vi "ge_PopGlobals.vi"(8 "error in":errorcluster, 9 "Selected Rows":i32[](array[numeric]), 10 "ChanGrp.lvclass":refnum<class "ChanGrp.lvclass">, 11 "ge_DAQManDefinitions":T1) -> (0 "error out":errorcluster, 1 "DefVal":u16=65535, 3 "Ring Support For Group":variant)   [LabVIEW 2012]
uses:
  Classes/Cfg Grandmaster/Class Chan Group/ChanGrp.lvclass
  Common/Controls/DAQMan Definitions.ctl
  Classes/Cfg Grandmaster/Class Chan Group/Read MeasType.vi
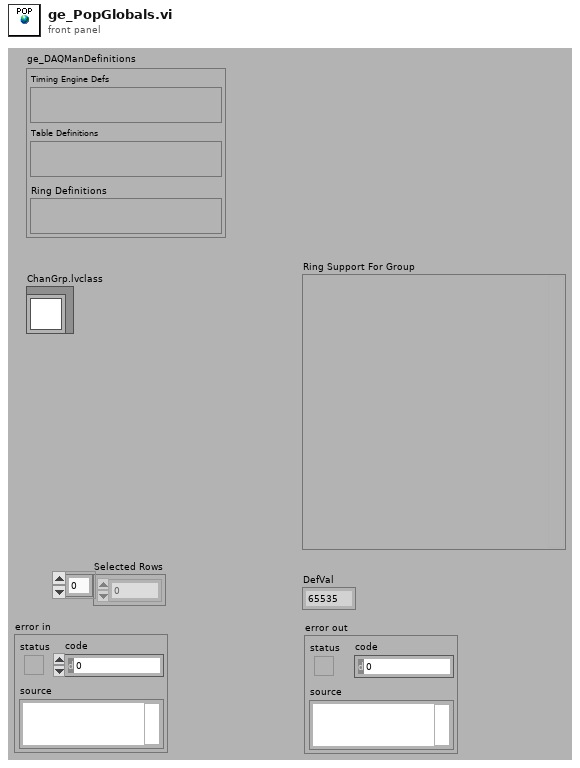
[diagram p1: front panel]
types:
  T1 = typedef "DAQMan Definitions.ctl" = cluster{"Timing Engine Defs":variant, "Table Definitions":variant, "Ring Definitions":variant}
  T2 = typedef "ge_MeasType.ctl" = enum16{"Voltage", "Frequency", "Tachometer", "Dynamic", "Thermocouple", "RTD", "Strain", "Current", "Resistance"}
  T3 = typedef "HeaderNames.ctl" = enum16{"Channel", "Device", "Spacer", "Description", "MB", "Range", "Terminal", "Coupling", "Thresh (V)", "Pulse/Rev", "Slope", "Min EU", "Min RPM", "mV/EU", "Iex", "Temp Units", "Type", "CJC Src", "CJC Val", "Ro", "Wire Cfg", "Strain Mode", "Vex", "Bridge Type", "GF", "Gauge Res", "Poisson", "Lead Res", "Init Strain", "GAF", "Scale", "Offset", "Unit (EU)", "dB?", "dB Ref", "Cal Mag", "Cal Units", "Max Temp", "Min Temp", "Max Strain", "Min Strain"}
  T4 = typedef "ge_StringVals.ctl" = cluster{"String":string, "Value":u16}
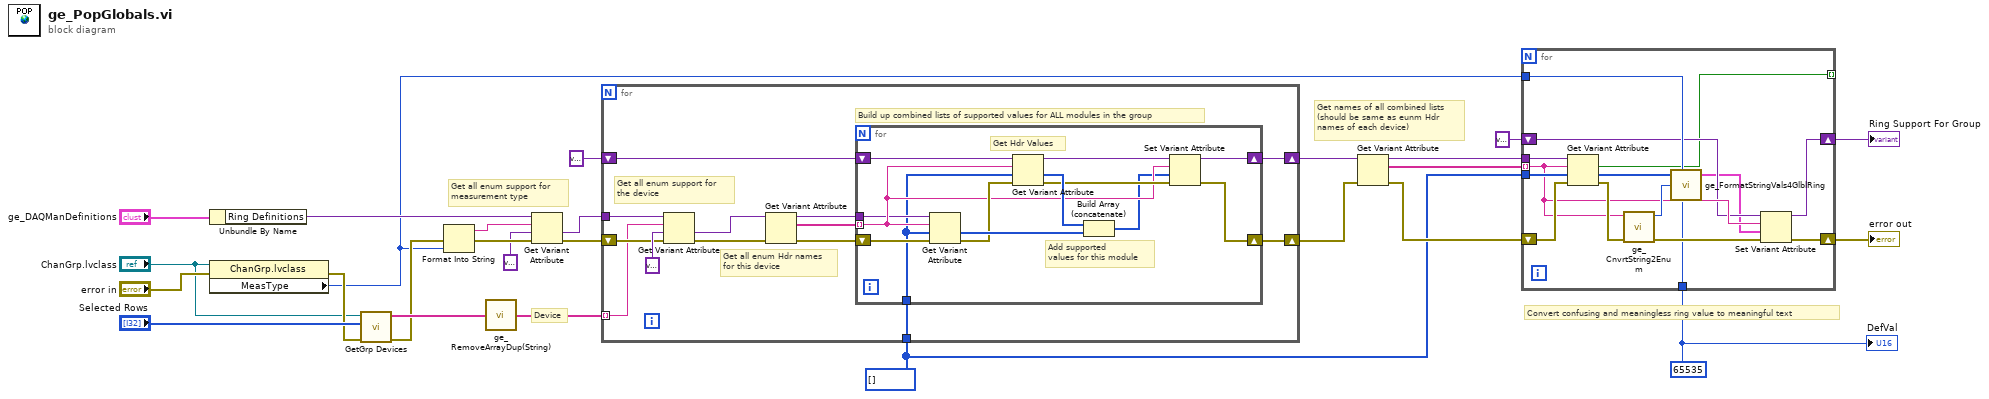
[diagram p0: block diagram]
diagram:
  w8 = u16 65535 ("DefVal")
  w12 = u16[] [] ("Values")
  # "Convert confusing and meaningless ring value to meaningful text"
  # "Get names of all combined lists\n(should be same as eunm Hdr\nnames of each device)"
  # "Get all enum support for\nmeasurement type"
  # "Device"
  n1 = Unbundle By Name("ge_DAQManDefinitions") -> ("Ring Definitions"=w6:variant)
  n2 = property class="ChanGrp.lvclass"(reference="ChanGrp.lvclass", error in="error in") -> (error out=w5:errorcluster, "MeasType"=w1:T2)  [unwired: 1 out]
  n3 = call "GetGrp Devices.vi"("error in (no error)"=w5, "Selected Rows"="Selected Rows", "ChanGrp.lvclass"="ChanGrp.lvclass") -> ("error out"=w2:errorcluster, "Dev Array"=w24:string[])  [unwired: 7 in]
  n4 = Format Into String(error in=w2, w1) -> (resulting string=w22:string, error out=w23:errorcluster)  [unwired: 2 in]
  n5 = call "ge_RemoveArrayDup(String).vi"("Input Array"=w24) -> ("Output Array"=w25:string[])  [unwired: 4 in]
  n6 = Get Variant Attribute(Variant=w6, name=w22, default value (empty Variant)=variant ("All Ring Support"), error in=w23) -> (value=w20:variant, error out=w19:errorcluster)  [unwired: 2 out]
  n7 = for {
    tunnel: w25 -> [w32] mode=indexing
    tunnel: w20 -> [w38]
    shift-right: [w30] -> w16
    shift-left: w19 -> [w35]
    shift-right: [w29] -> w17
    shift-left: variant ("All Ring Support") -> [w31]
    tunnel: w12 -> [w27]
    # "Build up combined lists of supported values for ALL modules in the group"
    # "Get all enum support for\nthe device"
    # "Get all enum Hdr names\nfor this device"
    n8 = Get Variant Attribute(Variant=w38, name=w32, default value (empty Variant)=variant ("All Ring Support"), error in=w35) -> (value=w34:variant, error out=w37:errorcluster)  [unwired: 2 out]
    n9 = Get Variant Attribute(Variant=w34, error in=w37) -> (duplicate Variant=w28:variant, names=w36:string[], error out=w33:errorcluster)  [unwired: 2 in, 1 out]
    n10 = for {
      shift-right: [w52] -> w29
      shift-left: w31 -> [w49]
      tunnel: w36 -> [w43] mode=indexing
      shift-right: [w44] -> w30
      shift-left: w33 -> [w51]
      tunnel: w28 -> [w41]
      tunnel: w27 -> [w40]
      # "Add supported\nvalues for this module"
      # "Get Hdr Values"
      n11 = Get Variant Attribute(Variant=w41, name=w43, default value (empty Variant)=w40, error in=w51) -> (value=w50:u16[], error out=w47:errorcluster)  [unwired: 2 out]
      n12 = Get Variant Attribute(Variant=w49, name=w43, default value (empty Variant)=w40, error in=w47) -> (duplicate Variant=w48:variant, value=w46:u16[], error out=w45:errorcluster)  [unwired: 1 out]
      n13 = Build Array (concatenate)(w46, w50) -> (w42:u16[])
      n14 = Set Variant Attribute(Variant=w48, name=w43, value=w42, error in=w45) -> (Variant out=w52:variant, error out=w44:errorcluster)  [unwired: 1 out]
    }
  }
  n15 = Get Variant Attribute(Variant=w17, error in=w16) -> (duplicate Variant=w15:variant, names=w14:string[], error out=w13:errorcluster)  [unwired: 2 in, 1 out]
  n16 = for {
    tunnel: w1 -> [w62]
    tunnel: w15 -> [w67]
    tunnel: w14 -> [w60] mode=indexing
    shift-right: [w59] -> w10
    shift-left: w13 -> [w66]
    tunnel: w12 -> [w65]
    shift-right: [w57] -> w9
    shift-left: variant ("All Ring Support") -> [w58]
    tunnel: [w56] -> _ mode=indexing
    tunnel: w8 -> [w53]
    n17 = Get Variant Attribute(Variant=w67, name=w60, default value (empty Variant)=w65, error in=w66) -> (found=w56:bool, value=w55:u16[], error out=w64:errorcluster)  [unwired: 1 out]
    n18 = call "ge_CnvrtString2Enum.vi"("error in (no error)"=w64, "Enum String"=w60) -> ("error out"=w63:errorcluster, "Hdr Name"=w61:T3)  [unwired: 8 in]
    n19 = call "ge_FormatStringVals4GlblRing.vi"("Values"=w55, "MeasType"=w62, "Hdr Name"=w61, "DefVal"=w53) -> ("String and Values"=w54:T4[])  [unwired: 3 in]
    n20 = Set Variant Attribute(Variant=w58, name=w60, value=w54, error in=w63) -> (Variant out=w57:variant, error out=w59:errorcluster)  [unwired: 1 out]
  }
  "error out" <- w10
  "Ring Support For Group" <- w9
  "DefVal" <- w8
